vi "arrays.vi"() -> ()   [LabVIEW 2020]
panel:
  out "1,2":i32
  out "2":i32[](array[numeric])
  out "1":i32[](array[numeric])
  out "Elemento posicion 2":i32
  out "Concatenaded input":i32[](array[numeric])
  out "Appended array":i32[][](array[numeric])
  out "appended array":i32[](array[numeric])
  out "Areglo 2D subset":dbl[][](array[numeric])
  out "subarray":dbl[](array[numeric])
  out "Arreglo creado 2d automatico":dbl[][](array[numeric])
  out "Arreglo creado automatico":dbl[](array[numeric])
  out "Tamaño arreglo":i32[](array[numeric])
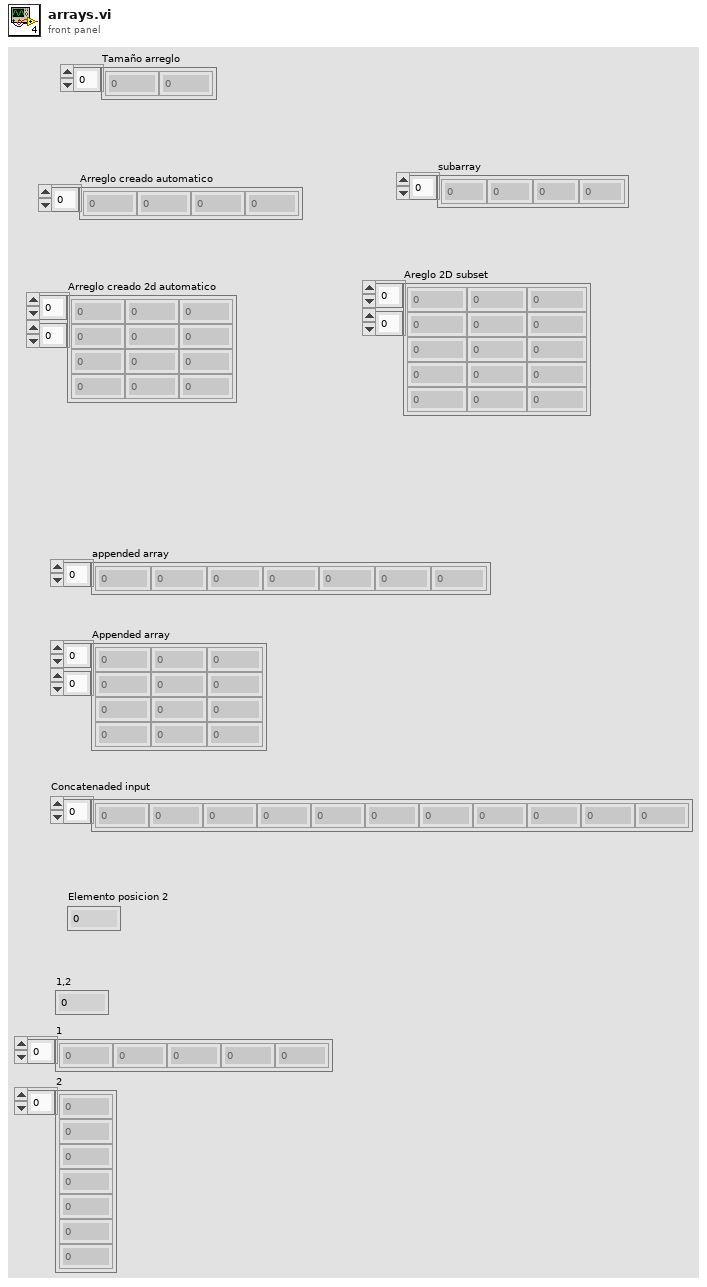
[diagram p1: front panel]
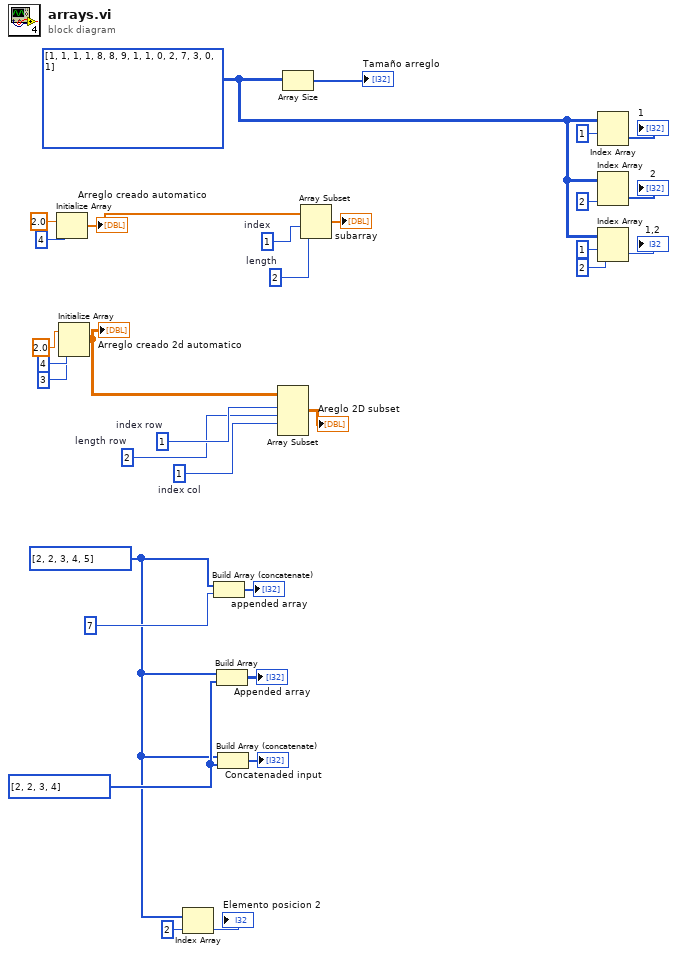
[diagram p0: block diagram]
diagram:
  w13 = i32[] [2, 2, 3, 4]
  w11 = i32[] [2, 2, 3, 4, 5]
  w17 = 2  # length row
  w19 = 1  # index col
  w20 = 1  # index row
  w23 = 2  # length
  w24 = 1  # index
  w8 = i32[][] [[1, 1, 1], [1, 8, 8], [9, 1, 1], [0, 2, 7], [3, 0, 1]]
  n1 = Initialize Array(2.0 ("element"), 4 ("dimension size")) -> (w25:dbl[])
  "Arreglo creado automatico" <- w25
  n2 = Initialize Array(2.0 ("element"), 4 ("dimension size"), 3 ("dimension size")) -> (w21:dbl[][])
  "Arreglo creado 2d automatico" <- w21
  n3 = Index Array(array=w11, index=2) -> (element=→"Elemento posicion 2":i32)
  n4 = Build Array (concatenate)(w11, 7) -> (→"appended array":i32[])
  n5 = Build Array(w11, w13) -> (→"Appended array":i32[][])
  n6 = Build Array (concatenate)(w11, w13) -> (→"Concatenaded input":i32[])
  n7 = Array Subset(array=w21, index (row)=w20, length (row)=w17, index (col)=w19) -> (→"Areglo 2D subset":dbl[][])  [unwired: 1 in]
  n8 = Array Size(array=w8) -> (size(s)=→"Tamaño arreglo":i32[])
  n9 = Array Subset(array=w25, index=w24, length=w23) -> (→"subarray":dbl[])
  n10 = Index Array(array=w8, index (row)=1) -> (element=→"1":i32[])  [unwired: 1 in]
  n11 = Index Array(array=w8, index (col)=2 ("disabled index (col)")) -> (element=→"2":i32[])  [unwired: 1 in]
  n12 = Index Array(array=w8, index (row)=1, index (col)=2 ("disabled index (col)")) -> (element=→"1,2":i32)
